vi "LSX Get Accel Func.vi"(0 "lLSID":i32, 1 "lR":i32, 5 "lX":i32, 7 "lY":i32, 9 "lZ":i32, 11 "error in (no error)":errorcluster) -> (3 "lR out":i32, 4 "function return":i32, 6 "lX out":i32, 8 "lY out":i32, 10 "lZ out":i32, 15 "error out":errorcluster)   [LabVIEW 2018, in "Tango.lvlib"]
doc: "TANGOAPI int TANGOCALL LSX_GetAccelFunc (int lLSID, int *lX, int *lY, int *lZ, int *lR);"
uses:
  <userlib>/Tango/Tango.lvlib
  <userlib>/Tango/Tango_DLL.dll
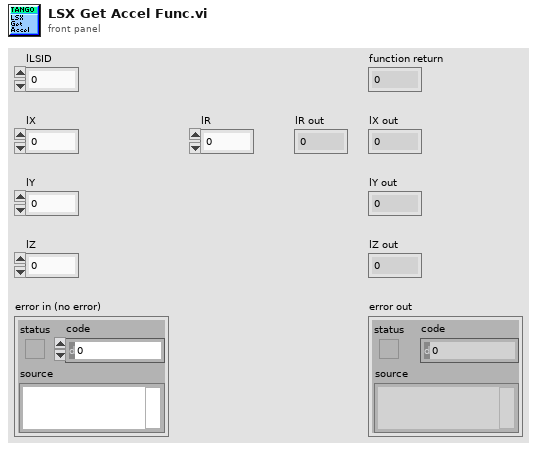
[diagram p1: front panel]
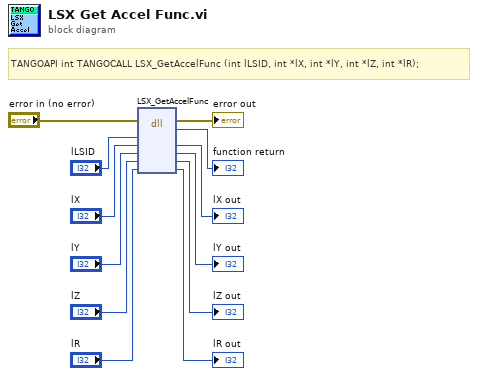
[diagram p0: block diagram]
diagram:
  # "TANGOAPI int TANGOCALL LSX_GetAccelFunc (int lLSID, int *lX, int *lY, int *lZ, int *lR);"
  n1 = dll-call lib="C:/Program Files (x86)/National Instruments/LabVIEW 2018/user.lib/Tango/Tango_DLL.*" fn="LSX_GetAccelFunc"(error in="error in (no error)", "lLSID"="lLSID", "lX"="lX", "lY"="lY", "lZ"="lZ", "lR"="lR") -> (error out=→"error out":errorcluster, →"function return":i32, "lX"=→"lX out":i32, "lY"=→"lY out":i32, "lZ"=→"lZ out":i32, "lR"=→"lR out":i32)  [unwired: 3 in, 1 out]
